vi "Scale Frequency from Freq.vi"(1 "Frequency":dbl[unit]=5000000.0) -> (0 "Frequency (scaled)":u32)   [LabVIEW 2009]
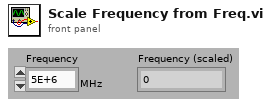
[diagram p1: front panel]
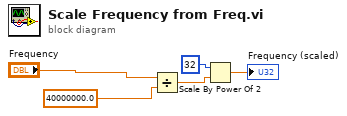
[diagram p0: block diagram]
diagram:
  n1 = Divide(x="Frequency", y=dbl[unit] 40000000.0) -> (x/y=w5:dbl)
  n2 = Scale By Power Of 2(n=i16 32, x=w5) -> (x*2^n=→"Frequency (scaled)":dbl)
